vi "Main.vi"() -> ()   [LabVIEW 2021]
doc: "Use this template to build a simple state machine design pattern. Each state executes code and determines which state to transition to."
uses:
  controls/State.ctl
  controls/Data.ctl
  <vilib>/DAQmx/configure/timing.llb/DAQmx Timing (Sample Clock).vi
  <vilib>/DAQmx/create/channels.llb/DAQmx Create Channel (AI-Voltage-Basic).vi
  <vilib>/Waveform/WDTOps.llb/WDT Append Waveforms DBL.vi
  <vilib>/DAQmx/read.llb/DAQmx Read (Analog Wfm 1Chan NSamp).vi
  <vilib>/daqmxs/DAQmx sim.lvlib
  <vilib>/daqmxs/DAQmx Read sim (Analog Wfm 1Chan NSamp).vi
  <vilib>/Utility/TDMS File Viewer/NI_TDMS File Viewer.lvlib
panel:
  out "Pocet period":i32
  out "Prubeh frekvence":waveform(dbl)(graph)
  in  "Hystereze":dbl min=0.0 step=0.1
  in  "Analyze data":bool
  in  "Threshold":dbl
  in  "Simulated signal":bool
  in  "Signal":refnum<k21>
  in  "stop measure":bool
  in  "Measure Init":bool
  in  "Number of Samples":i32=100
  in  "Sample Rate":dbl=1000.0
  in  "Sample Clock Source":tag="OnboardClock"
  in  "Terminal Configuration":i32(ring)=-1 items=["default"=-1, "RSE"=10083, "NRSE"=10078, "Differential"=10106, "Pseudodifferential"=12529]
  in  "Max Voltage":dbl=5.0
  in  "Min Voltage":dbl=-5.0
  in  "Physical Channel":tag="Dev1/ai0"
  out "Waveform Graph":waveform(dbl)(graph)
  in  "Write to TDMS":bool
  in  "Start measuring":bool
  in  "Exit":bool
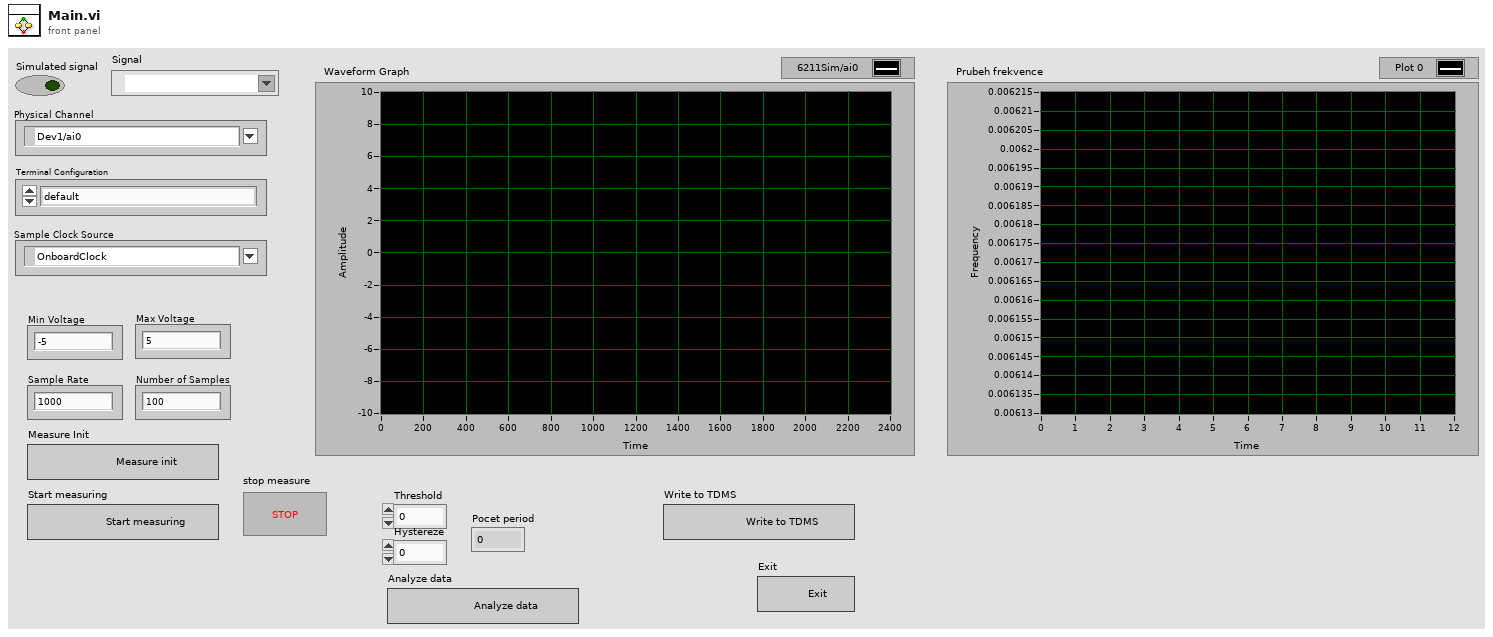
[diagram p1: front panel]
types:
  T1 = typedef "Data.ctl" = cluster{"DAQmx Task Name":refnum<k21>, "Mes running":bool, "Waveform":waveform(dbl), "Simulated signal":bool, "Pocet period":i32, "Prubeh frekvence":waveform(dbl)}
  T2 = typedef "State.ctl" = enum16{"Initialize", "Wait for Event", "Mesurement init", "START measure", "Measuring", "STOP measure", "Data analyze", "TDMS write", "Error", "Exit"}
  T3 = enum8{"Enabled", "Disabled", "Disabled and Grayed Out"}
  T4 = enum16{"open", "open or create", "create or replace", "create", "open (read-only)"}
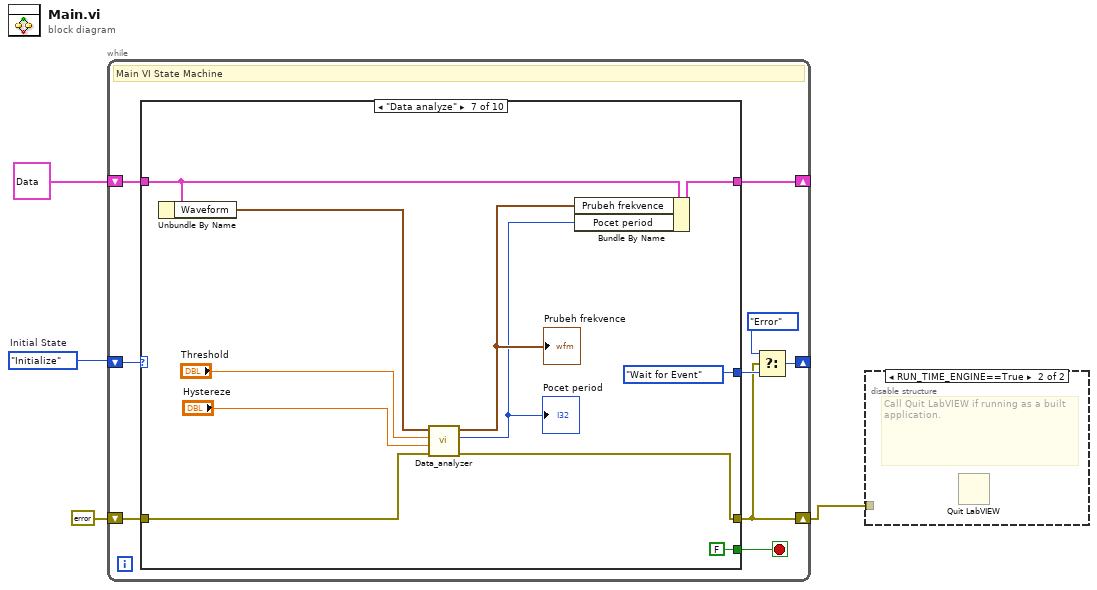
[diagram p0: block diagram]
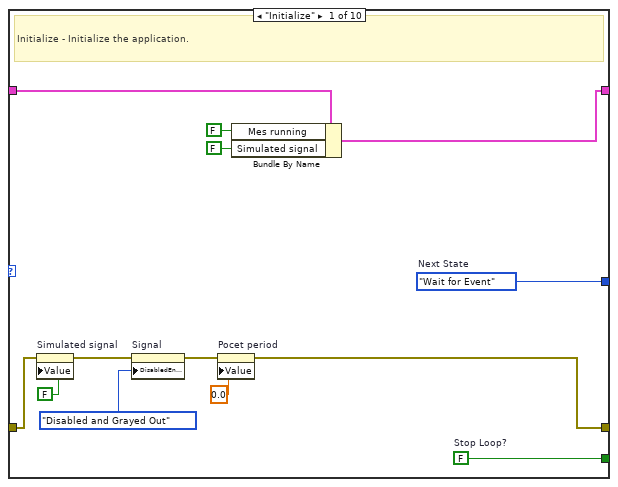
[diagram p3: hidden frame]
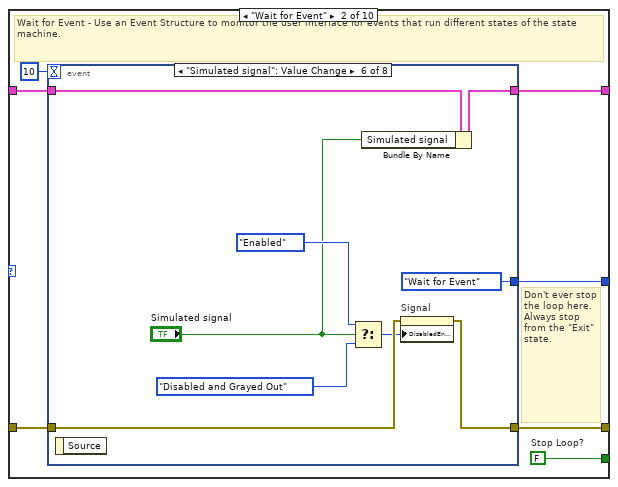
[diagram p4: hidden frame]
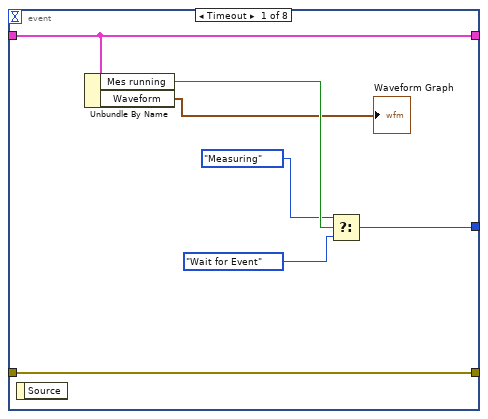
[diagram p5: hidden frame]
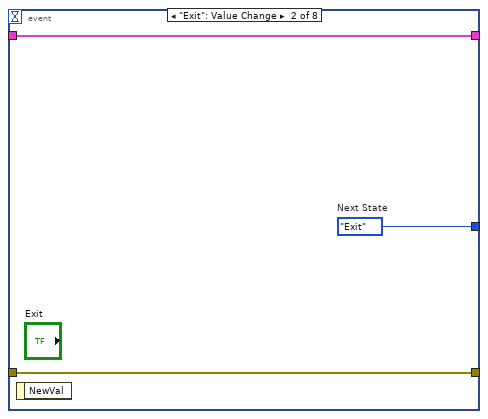
[diagram p6: hidden frame]
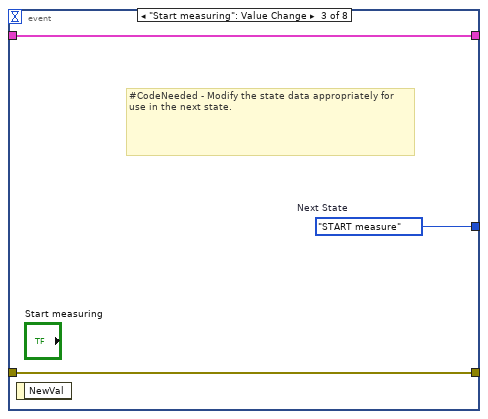
[diagram p7: hidden frame]
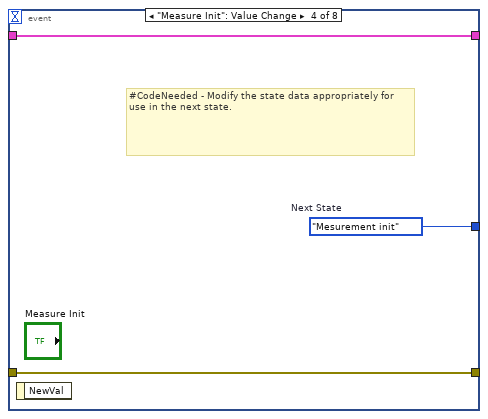
[diagram p8: hidden frame]
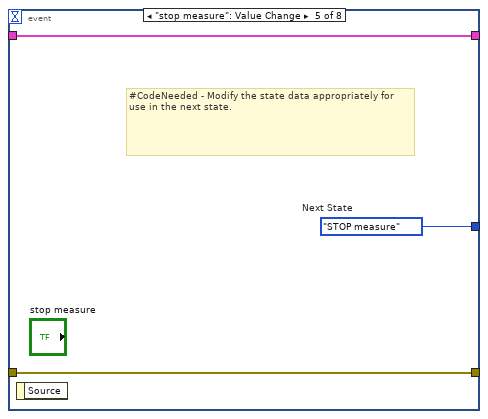
[diagram p9: hidden frame]
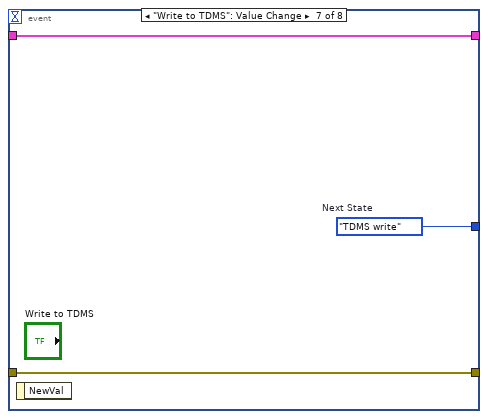
[diagram p10: hidden frame]
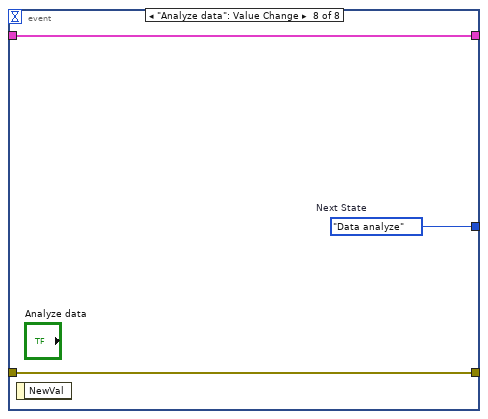
[diagram p11: hidden frame]
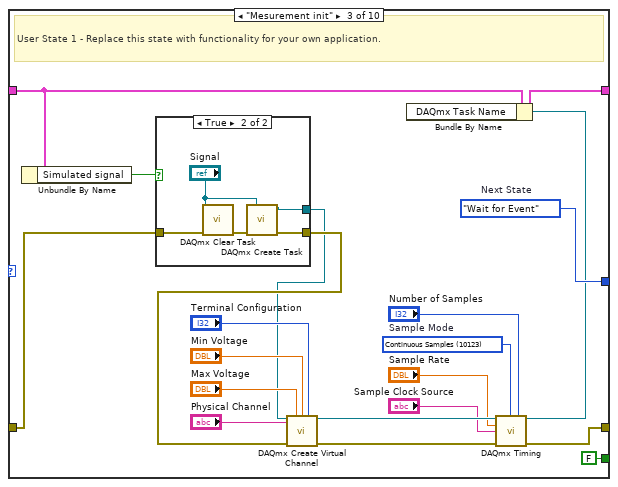
[diagram p12: hidden frame]
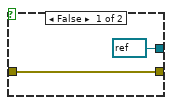
[diagram p13: hidden frame]
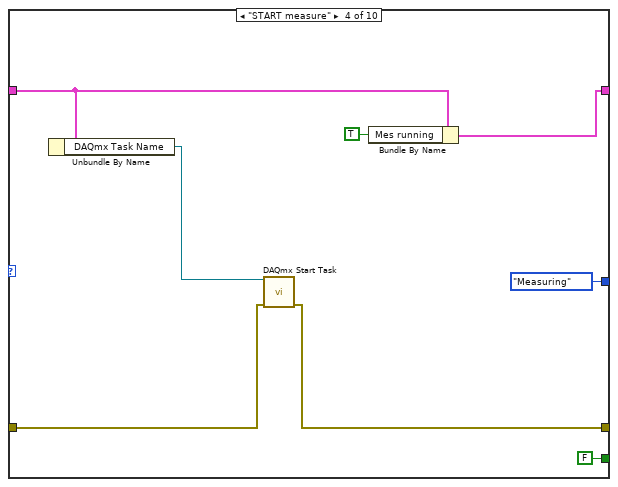
[diagram p14: hidden frame]
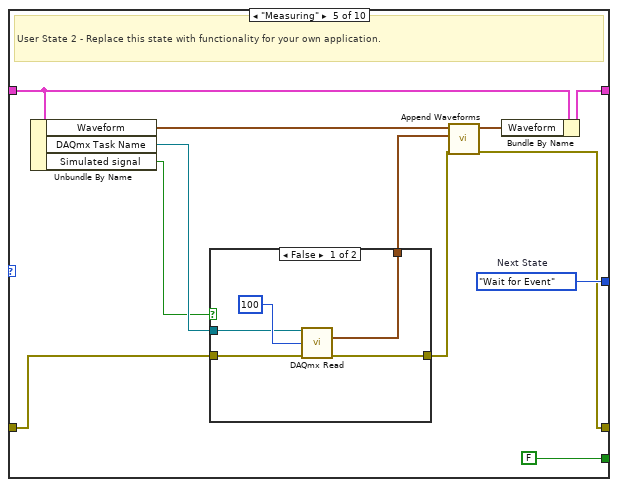
[diagram p15: hidden frame]
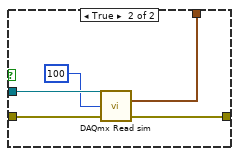
[diagram p16: hidden frame]
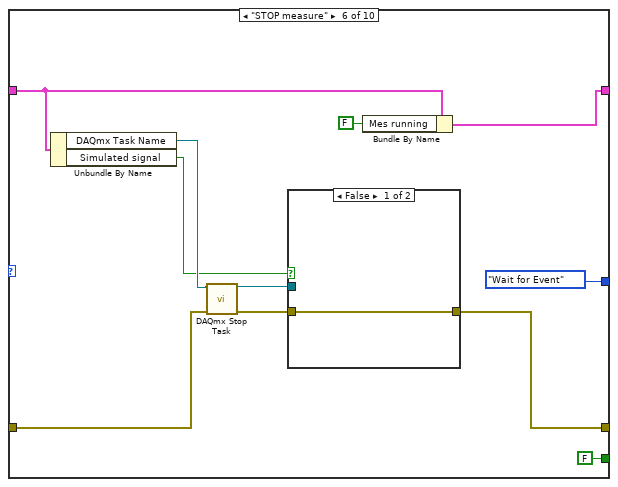
[diagram p17: hidden frame]
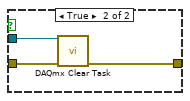
[diagram p18: hidden frame]
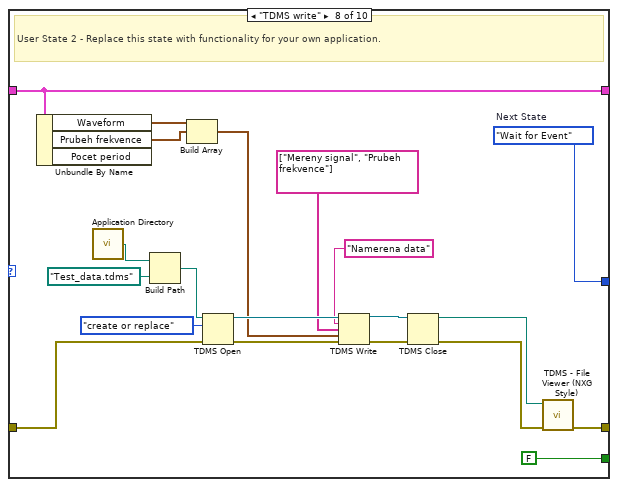
[diagram p19: hidden frame]
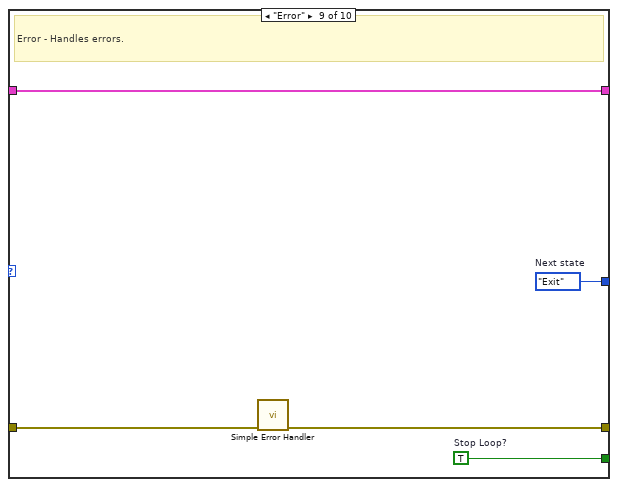
[diagram p20: hidden frame]
diagram:
  w2 = State."Initialize"  # Initial State
  n1 = while {
    shift-right: [w7] -> _
    shift-left: w2 -> [w13]
    shift-right: [w11] -> _
    shift-left: T1 {"DAQmx Task Name"="", "Mes running"=FALSE, "Waveform"={"t0"=timestamp(0 s since 1904-01-01), "dt"=1.0, "Y"=[]}, "Simulated signal"=FALSE, "Pocet period"=0, "Prubeh frekvence"={"t0"=timestamp(0 s since 1904-01-01), "dt"=1.0, "Y"=[]}} ("Data") -> [w12]
    shift-right: [w5] -> w1
    shift-left: errorcluster {"status"=FALSE, "code"=0, "source"=""} ("error constant") -> [w10]
    stop <- w9 stop-if-true
    # "Main VI State Machine"
    n2 = case shown="\"Data analyze\"" w13 {
      tunnel: [w26 w33 w87 State."Measuring" ("Next state") w114 State."Wait for Event" ("Next state") State."Wait for Event" ("Next state") w170 w175 w181] -> w8
      tunnel: [w25 w32 FALSE ("Stop Loop?") FALSE ("Stop Loop?") FALSE ("Stop Loop?") FALSE ("Stop Loop?") FALSE ("Stop Loop?") FALSE ("Stop Loop?") w173 w180] -> w9
      tunnel: w12 -> [w24 w31 w69 w97 w105 w133 w143 w168 w174 w177]
      tunnel: [w23 w30 w85 w96 w111 w132 w142 w168 w174 w177] -> w11
      tunnel: w10 -> [w19 w29 w72 w102 w112 w129 w148 w158 w172 w179]
      tunnel: [w14 w28 w74 w101 w107 w126 w147 w167 w171 w178] -> w5
      frame "Initialize" {
        w25 = FALSE  # Stop Loop?
        w26 = State."Wait for Event"  # Next State
        # "Initialize - Initialize the application."
        n3 = property on="Simulated signal" class="Bool (strict)"(error in=w19, "Value"=FALSE ("Simulated device")) -> (error out=w18:errorcluster)  [unwired: 1 in, 1 out]
        n4 = property on="Signal" class="DAQmxName (strict)"(error in=w18, "DisabledEnum"=T3."Disabled and Grayed Out" ("Disabled")) -> (error out=w16:errorcluster)  [unwired: 1 in, 1 out]
        n5 = property on="Pocet period" class="DigNum (strict)"(error in=w16, "Value"=0.0 ("Pocet period")) -> (error out=w14:errorcluster)  [unwired: 1 in, 1 out]
        n6 = Bundle By Name(cluster=w24, "Mes running"=FALSE, "Simulated signal"=FALSE ("Simulated device")) -> (w23:T1)
      }
      frame "Wait for Event" {
        w32 = FALSE  # Stop Loop?
        # "Don't ever stop the loop here. Always stop from the \"Exit\" state."
        # "Wait for Event - Use an Event Structure to monitor the user interface for events that run different states of the state machine."
        n7 = event shown="[5] \"Simulated signal\": Value Change" {
          selector: _ -> [_ _ _ _ _ _ _ _]
          dyn-events: _ -> [_ _ _ _ _ _ _ _]
          timeout: 10 -> [_ _ _ _ _ _ _ _]
          tunnel: [w39 w43 w46 w49 w52 State."Wait for Event" ("Next State") w64 w67] -> w33
          tunnel: w31 -> [w38 w42 w44 w47 w50 w55 w62 w65]
          tunnel: [w38 w42 w44 w47 w50 w54 w62 w65] -> w30
          tunnel: w29 -> [w40 w41 w45 w48 w51 w61 w63 w66]
          tunnel: [w40 w41 w45 w48 w51 w60 w63 w66] -> w28
          event Timeout {
            n8 = event-data() -> ()  [unwired: 1 in, 1 out]
            n9 = Unbundle By Name(w38) -> ("Mes running"=w37:bool, "Waveform"=→"Waveform Graph":waveform(dbl))
            n10 = Select(t=State."Measuring" ("Next State"), s=w37, f=State."Wait for Event" ("Next State")) -> (s? t:f=w39:T2)
          }
          event "Exit": Value Change {
            w43 = State."Exit"  # Next State
            n11 = event-data() -> ()  [unwired: 1 in, 1 out]
          }
          event "Start measuring": Value Change {
            w46 = State."START measure"  # Next State
            # "#CodeNeeded - Modify the state data appropriately for use in the next state."
            n12 = event-data() -> ()  [unwired: 1 in, 1 out]
          }
          event "Measure Init": Value Change {
            w49 = State."Mesurement init"  # Next State
            # "#CodeNeeded - Modify the state data appropriately for use in the next state."
            n13 = event-data() -> ()  [unwired: 1 in, 1 out]
          }
          event "stop measure": Value Change {
            w52 = State."STOP measure"  # Next State
            # "#CodeNeeded - Modify the state data appropriately for use in the next state."
            n14 = event-data() -> ()  [unwired: 1 in, 1 out]
          }
          event "Simulated signal": Value Change {
            n15 = event-data() -> ()  [unwired: 1 in, 1 out]
            n16 = Select(t=T3."Enabled" ("Disabled"), s="Simulated signal", f=T3."Disabled and Grayed Out" ("Disabled")) -> (s? t:f=w59:T3)
            n17 = Bundle By Name(cluster=w55, "Simulated signal"="Simulated signal") -> (w54:T1)
            n18 = property on="Signal" class="DAQmxName (strict)"(error in=w61, "DisabledEnum"=w59) -> (error out=w60:errorcluster)  [unwired: 1 in, 1 out]
          }
          event "Write to TDMS": Value Change {
            w64 = State."TDMS write"  # Next State
            n19 = event-data() -> ()  [unwired: 1 in, 1 out]
          }
          event "Analyze data": Value Change {
            w67 = State."Data analyze"  # Next State
            n20 = event-data() -> ()  [unwired: 1 in, 1 out]
          }
        }
      }
      frame "Mesurement init" {
        w84 = 10123 items=["Finite Samples"=10178, "Continuous Samples"=10123, "Hardware Timed Single Point"=12522]  # Sample Mode
        w87 = State."Wait for Event"  # Next State
        # "User State 1 - Replace this state with functionality for your own application."
        n21 = Unbundle By Name(w69) -> ("Simulated signal"=w68:bool)
        n22 = case shown="True" w68 {
          tunnel: w72 -> [w89 w92]
          tunnel: [w89 w91] -> w71
          tunnel: [refnum<k21> refnum ("task out") w90] -> w70
          frame False {
          }
          frame True {
            n23 = call <vilib>:"DAQmx Clear Task.vi"("task in"="Signal", "error in"=w92) -> ("error out"=w94:errorcluster)  [unwired: 13 in]
            n24 = call <vilib>:"DAQmx Create Task.vi"("new task name"="Signal", "error in"=w94) -> ("task out"=w90:refnum<k21>, "error out"=w91:errorcluster)  [unwired: 12 in]
          }
        }
        n25 = call-poly <vilib>:"DAQmx Create Virtual Channel.vi"("task in"=w70, "maximum value"="Max Voltage", "minimum value"="Min Voltage", "input terminal configuration"="Terminal Configuration", "physical channels"="Physical Channel", "error in"=w71) -> ("task out"=w82:refnum<k21>, "error out"=w83:errorcluster)  [unwired: 8 in]
        n26 = call-poly <vilib>:"DAQmx Timing.vi"("task/channels in"=w82, "sample mode"=w84, "samples per channel"="Number of Samples", "rate"="Sample Rate", "source"="Sample Clock Source", "error in"=w83) -> ("task out"=w73:refnum<k21>, "error out"=w74:errorcluster)  [unwired: 8 in]
        n27 = Bundle By Name(cluster=w69, "DAQmx Task Name"=w73) -> (w85:T1)
      }
      frame "START measure" {
        n28 = Unbundle By Name(w97) -> ("DAQmx Task Name"=w100:refnum<k21>)
        n29 = call <vilib>:"DAQmx Start Task.vi"("task/channels in"=w100, "error in"=w102) -> ("error out"=w101:errorcluster)  [unwired: 12 in, 1 out]
        n30 = Bundle By Name(cluster=w97, "Mes running"=TRUE) -> (w96:T1)
      }
      frame "Measuring" {
        w114 = State."Wait for Event"  # Next State
        # "User State 2 - Replace this state with functionality for your own application."
        n31 = Unbundle By Name(w105) -> ("Waveform"=w110:waveform(dbl), "DAQmx Task Name"=w104:refnum<k21>, "Simulated signal"=w103:bool)
        n32 = case shown="False" w103 {
          tunnel: w112 -> [w119 w124]
          tunnel: [w117 w123] -> w108
          tunnel: [w116 w120] -> w106
          tunnel: w104 -> [w115 w122]
          frame False {
            n33 = call-poly <vilib>:"DAQmx Read.vi"("task/channels in"=w115, "number of samples per channel"=100, "error in"=w119) -> ("data"=w116:waveform(dbl), "error out"=w117:errorcluster)  [unwired: 10 in, 1 out]
          }
          frame True {
            n34 = call-poly <vilib>:"DAQmx Read sim.vi"("task/channels in"=w122, "number of samples per channel"=100, "error in"=w124) -> ("data"=w120:waveform(dbl), "error out"=w123:errorcluster)  [unwired: 10 in, 1 out]
          }
        }
        n35 = call-poly <vilib>:"Append Waveforms.vi"("error in (no error)"=w108, "waveform B"=w106, "waveform A"=w110) -> ("error out"=w107:errorcluster, "waveform out"=w109:waveform(dbl))  [unwired: 7 in]
        n36 = Bundle By Name(cluster=w105, "Waveform"=w109) -> (w111:T1)
      }
      frame "STOP measure" {
        n37 = Unbundle By Name(w133) -> ("DAQmx Task Name"=w130:refnum<k21>, "Simulated signal"=w125:bool)
        n38 = call <vilib>:"DAQmx Stop Task.vi"("task/channels in"=w130, "error in"=w129) -> ("task out"=w127:refnum<k21>, "error out"=w128:errorcluster)  [unwired: 12 in]
        n39 = case shown="False" w125 {
          tunnel: w128 -> [w136 w139]
          tunnel: w127 -> [_ w138]
          tunnel: [w136 w137] -> w126
          frame False {
          }
          frame True {
            n40 = call <vilib>:"DAQmx Clear Task.vi"("task in"=w138, "error in"=w139) -> ("error out"=w137:errorcluster)  [unwired: 13 in]
          }
        }
        n41 = Bundle By Name(cluster=w133, "Mes running"=FALSE) -> (w132:T1)
      }
      frame "Data analyze" {
        n42 = Unbundle By Name(w143) -> ("Waveform"=w144:waveform(dbl))
        n43 = call "Data_analyzer.vi"("error in"=w148, "Hystereze"="Hystereze", "Uroven mereni"="Threshold", "Data"=w144) -> ("error out"=w147:errorcluster, "Pocet period"=w140:i32, "Prubeh frekvence"=w141:waveform(dbl))  [unwired: 5 in]
        "Prubeh frekvence" <- w141
        "Pocet period" <- w140
        n44 = Bundle By Name(cluster=w143, "Prubeh frekvence"=w141, "Pocet period"=w140) -> (w142:T1)
      }
      frame "TDMS write" {
        w170 = State."Wait for Event"  # Next State
        # "User State 2 - Replace this state with functionality for your own application."
        n45 = Unbundle By Name(w168) -> ("Waveform"=w157:waveform(dbl), "Prubeh frekvence"=w156:waveform(dbl))  [unwired: 1 out]
        n46 = call <vilib>:"Application Directory.vi"() -> ("Application Directory"=w162:path)
        n47 = Build Path(base path=w162, name or relative path=path "Test_data.tdms") -> (appended path=w160:path)
        n48 = Build Array(w157, w156) -> (w155:waveform(dbl)[])  [unwired: 1 in]
        n49 = TDMS Open(8:w158, 10:T4."create or replace" ("operation (0:open)"), 11:w160) -> (0:w164:errorcluster, 3:w163:refnum<k34>)  [unwired: 4 in]
        n50 = TDMS Write(0:w163, 5:"Namerena data" ("group name in (Untitled)"), 7:string[] ["Mereny signal", "Prubeh frekvence"] ("channel name(s) in (Untitled)"), 9:w155, 11:w164) -> (4:w165:refnum<k34>, 15:w166:errorcluster)  [unwired: 1 in, 2 out]
        n51 = TDMS Close(8:w166, 11:w165) -> (0:w152:errorcluster, 3:w151:path)
        n52 = call <vilib>:"TDMS - File Viewer (NXG Style).vi"("error in"=w152, "file in"=w151) -> ("error out"=w167:errorcluster)  [unwired: 8 in, 1 out]
      }
      frame "Error" {
        w173 = TRUE  # Stop Loop?
        w175 = State."Exit"  # Next state
        # "Error - Handles errors."
        n53 = call <vilib>:"Simple Error Handler.vi"("error in (no error)"=w172) -> ("error out"=w171:errorcluster)  [unwired: 4 in, 4 out]
      }
      frame "Exit" {
        w180 = TRUE  # Stop Loop?
        w181 = State."Exit"  # (Value Not Used)
        # "Exit - Exit the application."
        n54 = Unbundle By Name(w177) -> ("DAQmx Task Name"=w176:refnum<k21>)
        n55 = call <vilib>:"DAQmx Clear Task.vi"("task in"=w176, "error in"=w179) -> ("error out"=w178:errorcluster)  [unwired: 13 in]
      }
    }
    n56 = Select(t=State."Error", s=w5, f=w8) -> (s? t:f=w7:T2)
  }
  n57 = disable-structure shown="RUN_TIME_ENGINE==True" {
    disable-tunnel: w1 -> [_ _]
    frame condition #0 (active) {
    }
    frame condition #1 {
      # "Call Quit LabVIEW if running as a built application."
      n58 = Quit LabVIEW() -> ()  [unwired: 1 in]
    }
  }
